vi "turn_.vi"(9 "delay":u32, 10 "Carzeta":dbl) -> ()   [LabVIEW 2017]
uses:
  GlobalVar.vi
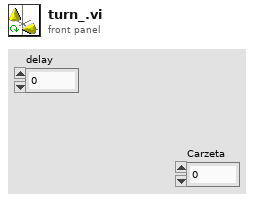
[diagram p1: front panel]
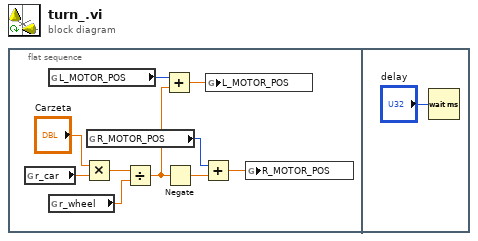
[diagram p0: block diagram]
diagram:
  n1 = flat-sequence {
    frame #0 {
      n2 = global read "GlobalVar.vi" "r_car"() -> (w3:dbl)
      n3 = global read "GlobalVar.vi" "L_MOTOR_POS"() -> (w8:i32)
      n4 = global read "GlobalVar.vi" "r_wheel"() -> (w4:dbl)
      n5 = Multiply(x="Carzeta", y=w3) -> (x*y=w9:dbl)
      n6 = global read "GlobalVar.vi" "R_MOTOR_POS"() -> (w7:i32)
      n7 = Divide(x=w9, y=w4) -> (x/y=w1:dbl)
      n8 = Add(x=w8, y=w1) -> (x+y=w6:dbl)
      n9 = Negate(x=w1) -> (-x=w2:dbl)
      n10 = Add(x=w7, y=w2) -> (x+y=w5:dbl)
      n11 = global write "GlobalVar.vi" "L_MOTOR_POS"(w6) -> ()
      n12 = global write "GlobalVar.vi" "R_MOTOR_POS"(w5) -> ()
    }
    frame #1 {
      n13 = Wait (ms)(milliseconds to wait="delay") -> ()  [unwired: 1 out]
    }
  }
